vi "ChangePlotSize.vi"(8 "error in (no error)":errorcluster caption="错误输入（无错误）", 11 "XYPlot 输入":refnum<class "TrendPlot.lvclass">) -> (0 "error out":errorcluster caption="错误输出", 3 "XYPlot 输出":refnum<class "TrendPlot.lvclass">)   [LabVIEW 2018, in "DataDisplay.lvlib" / "TrendPlot.lvclass"]
uses:
  TrendPlot.lvclass
  <vilib>/Utility/miscctls.llb/LVBoundsTypeDef.ctl
  <vilib>/Utility/miscctls.llb/LVPositionTypeDef.ctl
  TrendPlot.lvclass/TrendPlot.ctl
panel:
  out "波形图":waveform(dbl)[](graph)
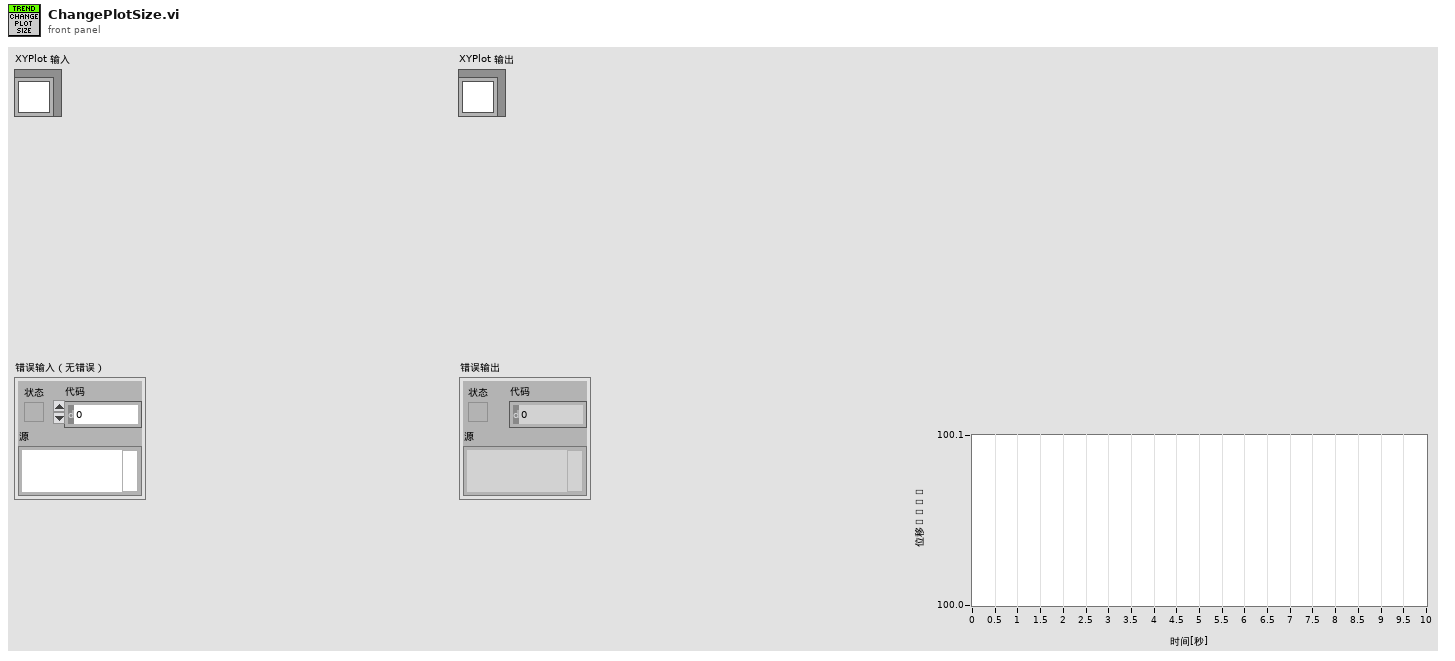
[diagram p1: front panel]
types:
  T1 = typedef "LVPositionTypeDef.ctl" = cluster{"Left":i32, "Top":i32}
  T2 = typedef "LVBoundsTypeDef.ctl" = cluster{"Width":u32, "Height":u32}
  T3 = typedef "LVRectTypeDef.ctl" = cluster{"Left":i16, "Top":i16, "Right":i16, "Bottom":i16}
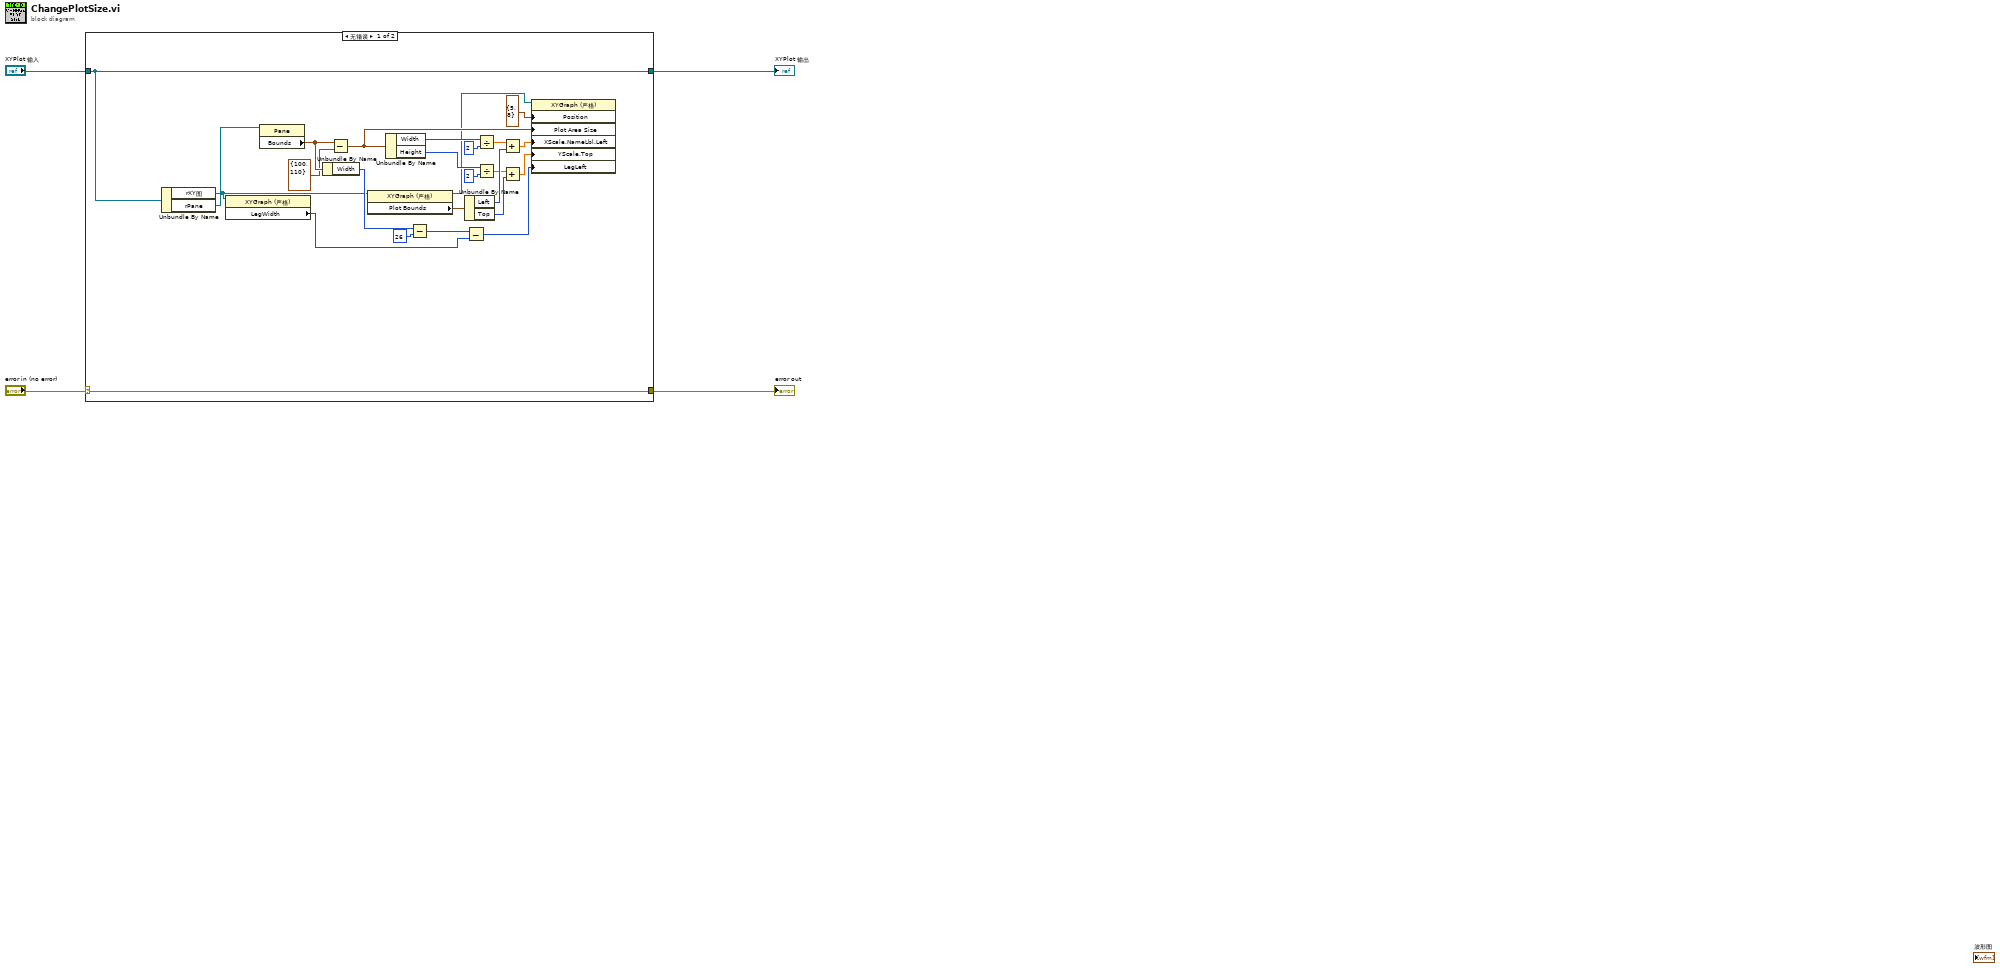
[diagram p0: block diagram]
diagram:
  n1 = case shown="无错误" "error in (no error)" {
    selector: "error in (no error)" -> [w29 w31]
    tunnel: [w29 w31] -> w3
    tunnel: [w28 w30] -> w1
    tunnel: "XYPlot 输入" -> [w28 w30]
    frame No Error {
      n2 = Unbundle By Name(w28) -> ("rXY图"=w6:refnum<vi>, "rPane"=w7:refnum<vi>)
      n3 = property class="XYGraph (严格)"(reference=w6) -> ("LegWidth"=w26:u32)  [unwired: 1 in, 2 out]
      n4 = property class="Pane"(reference=w7) -> ("Bounds"=w23:T2)  [unwired: 1 in, 2 out]
      n5 = Unbundle By Name(w23) -> ("Width"=w24:u32)
      n6 = Subtract(x=w23, y=T2 {"Width"=100, "Height"=110}) -> (x-y=w22:T2)
      n7 = property class="XYGraph (严格)"(reference=w6) -> (reference out=w12:refnum<vi>, "Plot Bounds"=w17:T3)  [unwired: 1 in, 1 out]
      n8 = Unbundle By Name(w22) -> ("Width"=w19:u32, "Height"=w21:u32)
      n9 = Subtract(x=w24, y=u32 26) -> (x-y=w25:u32)
      n10 = Unbundle By Name(w17) -> ("Left"=w18:i16, "Top"=w20:i16)
      n11 = Subtract(x=w25, y=w26) -> (x-y=w27:u32)
      n12 = Divide(x=w19, y=u32 2) -> (x/y=w13:dbl)
      n13 = Divide(x=w21, y=u32 2) -> (x/y=w15:dbl)
      n14 = Add(x=w13, y=w18) -> (x+y=w14:dbl)
      n15 = Add(x=w15, y=w20) -> (x+y=w16:dbl)
      n16 = property class="XYGraph (严格)"(reference=w12, "Position"=T1 {"Left"=5, "Top"=8} ("位置"), "Plot Area Size"=w22, "XScale.NameLbl.Left"=w14, "YScale.Top"=w16, "LegLeft"=w27) -> ()  [unwired: 1 in, 2 out]
    }
    frame Error {
    }
  }
  "error out" <- w3
  "XYPlot 输出" <- w1
